vi "CRC check.vi"(10 "array":u8[](array[numeric])) -> (2 "CRC":u16)   [LabVIEW 2023]
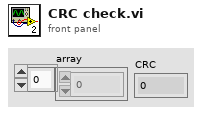
[diagram p1: front panel]
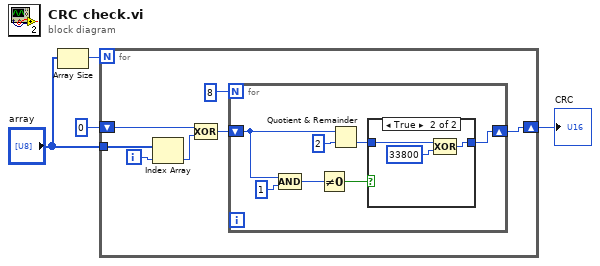
[diagram p0: block diagram]
diagram:
  n1 = Array Size(array="array") -> (size(s)=w4:i32)
  n2 = for {
    N: w4 -> [_]
    tunnel: "array" -> [w10]
    shift-right: [w5] -> w1
    shift-left: u8 0 -> [w7]
    i -> [w11]
    n3 = Index Array(array=w10, index=w11) -> (element=w9:u8)
    n4 = Compound Arithmetic op=XOR(w7, w9) -> (w6:u16)
    n5 = for {
      N: 8 -> [_]
      shift-right: [w12] -> w5
      shift-left: w6 -> [w15]
      n6 = Compound Arithmetic op=AND(w15, u8 1 ("value")) -> (w17:u16)
      n7 = Not Equal To 0?(x=w17) -> (x != 0?=w16:bool)
      n8 = Quotient & Remainder(x=w15, y=u8 2) -> (floor(x/y)=w13:u16)  [unwired: 1 out]
      n9 = case shown="True" w16 {
        tunnel: w13 -> [w19 w22]
        tunnel: [w19 w20] -> w12
        frame False {
        }
        frame True {
          n10 = Compound Arithmetic op=XOR(w22, u16 33800 ("value")) -> (w20:u16)
        }
      }
    }
  }
  "CRC" <- w1
